vi "9219_Is_TC_RTD.vi"(7 "Mode":i32) -> (6 "Is RIOScan / Thermocouple":bool, 8 "Is RIOScan / RTD":bool)   [LabVIEW 2020, in "Modules.lvlib" / "9219.lvclass"]
uses:
  9219.lvclass
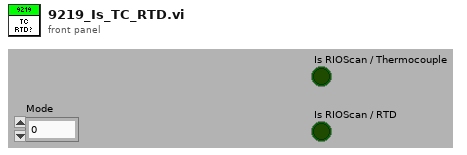
[diagram p1: front panel]
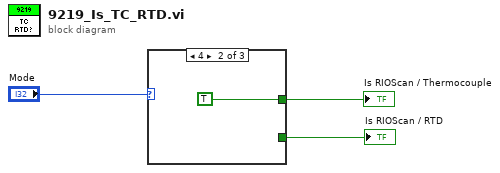
[diagram p0: block diagram]
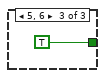
[diagram p3: hidden frame]
diagram:
  n1 = case shown="4" "Mode" {
    tunnel: [_ TRUE _] -> w3
    tunnel: [_ _ TRUE ("Is RIOScan / RTD")] -> w1
    frame Default {
    }
    frame 4 {
    }
    frame 5, 6 {
    }
  }
  "Is RIOScan / Thermocouple" <- w3
  "Is RIOScan / RTD" <- w1
